vi "Wait for modem AT cmd rdy.vi"(8 "error in (no error)":errorcluster, 11 "Open serial?":bool) -> (0 "error out":errorcluster={"status"=FALSE, "code"=1073676294, "source"="VISA Read in WaitForSpecificCommResponse.vi->Wait for sierra wireless ready.vi"}, 1 "timeout?":bool, 2 "Measurement":string, 3 "Elapsed time":string)   [LabVIEW 2013]
uses:
  Test Globals/Global 1.vi
panel:
  out "Secs loop":i32
  out "Elapsed time 2":dbl=3.480198860168457
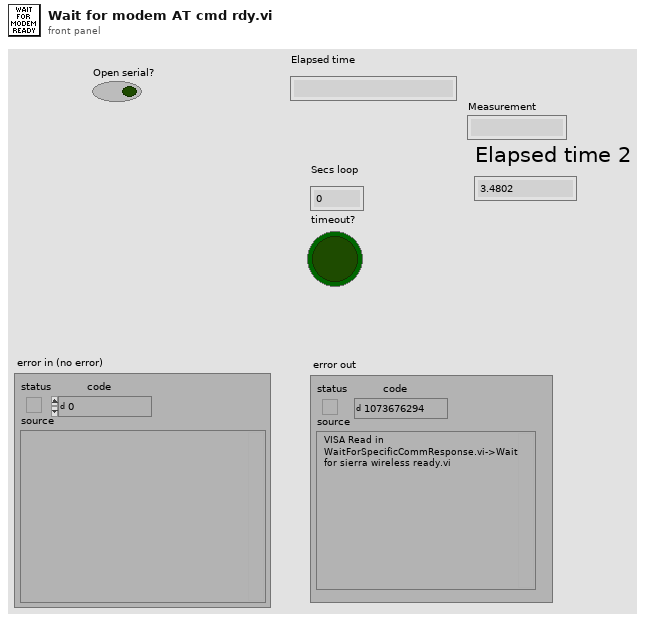
[diagram p1: front panel]
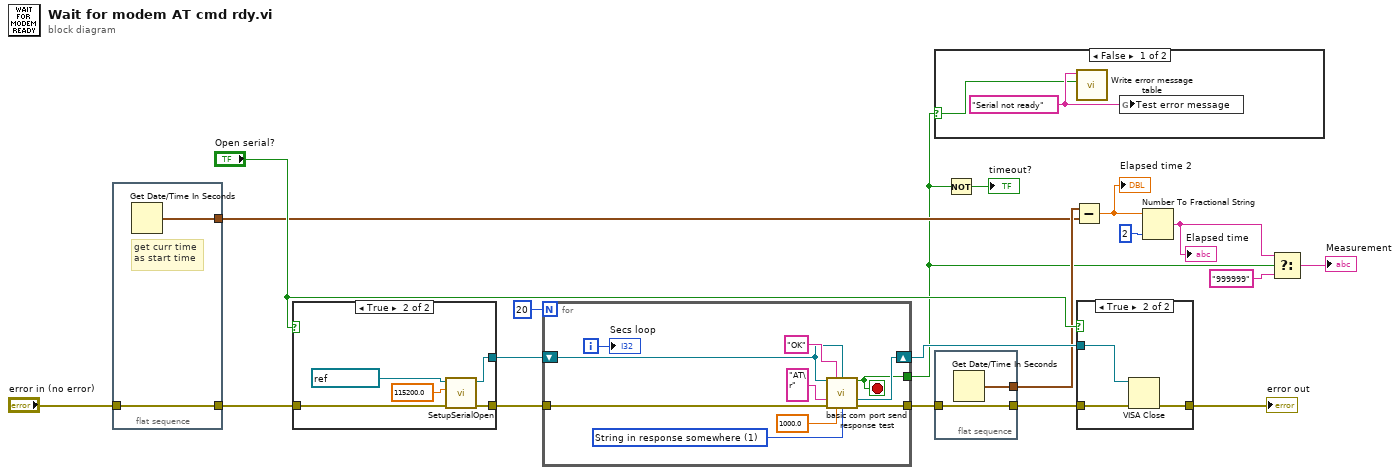
[diagram p0: block diagram]
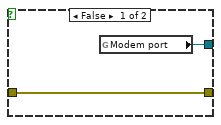
[diagram p4: hidden frame]
diagram:
  n1 = flat-sequence {
    tunnel: [w21] -> w5
    tunnel: "error in (no error)" -> [w20]
    tunnel: [w20] -> w7
    frame #0 {
      # "get curr time\nas start time"
      n2 = Get Date/Time In Seconds() -> (seconds since 1Jan1904=w21:timestamp)
    }
  }
  n3 = case shown="True" "Open serial?" {
    tunnel: w7 -> [w22 w26]
    tunnel: [w22 w25] -> w9
    tunnel: [w23 w24] -> w17
    frame False {
      n4 = global read "Global 1.vi" "Modem port"() -> (w23:refnum<visa-resource-name>)
    }
    frame True {
      n5 = call "SetupSerialOpen.vi"("error in (no error)"=w26, "Baud"=115200.0, "VISA Refnum in"=refnum<visa-resource-name> "COM30") -> ("error out"=w25:errorcluster, "VISA session"=w24:refnum<visa-resource-name>)  [unwired: 7 in]
    }
  }
  n6 = for {
    N: 20 -> [_]
    tunnel: w9 -> [w38]
    tunnel: [w33] -> w11
    tunnel: [w30] -> w2
    shift-right: [w31] -> w14
    shift-left: w17 -> [w32]
    i -> [w29]
    stop <- w30 stop-if-true
    w34 = u16 1 items=["String is exactly response", "String in response somewhere", "String not in response"] ("Comparison type")
    n7 = call "basic com port send response test.vi"("VISA Send port"=w32, "Expected response"="OK", "VISA Response Port"=w32, "Send text"="AT\r" ("write buffer"), "error in (no error)"=w38, "Wait for response msecs"=1000.0, "Comparison type"=w34) -> ("Response valid?"=w30:bool, "VISA Response Port out"=w31:refnum<visa-resource-name>, "error out"=w33:errorcluster)  [unwired: 4 in, 2 out]
    "Secs loop" <- w29
  }
  n8 = case shown="False" w2 {
    selector: w2 -> [w39 _]
    frame False {
      w40 = "Serial not ready" ("Error message)")
      n9 = call "Write error message table.vi"("Step passed?"=w39, "Error message)"=w40) -> ()  [unwired: 9 in, 1 out]
      n10 = global write "Global 1.vi" "Test error message"(w40) -> ()
    }
    frame True {
    }
  }
  n11 = flat-sequence {
    tunnel: w11 -> [w42]
    tunnel: [w42] -> w10
    tunnel: [w41] -> w6
    frame #0 {
      n12 = Get Date/Time In Seconds() -> (seconds since 1Jan1904=w41:timestamp)
    }
  }
  n13 = Not(x=w2) -> (.not. x?=→"timeout?":bool)
  n14 = Subtract(x=w6, y=w5) -> (x-y=w13:dbl)
  "Elapsed time 2" <- w13
  n15 = case shown="True" "Open serial?" {
    tunnel: [w43 w46] -> w16
    tunnel: w14 -> [_ w45]
    tunnel: w10 -> [w43 w44]
    frame False {
    }
    frame True {
      n16 = VISA Close(VISA resource name=w45, error in (no error)=w44) -> (error out=w46:errorcluster)
    }
  }
  "error out" <- w16
  n17 = Number To Fractional String(number=w13, precision (6)=i16 2) -> (F-format string=w4:string)  [unwired: 2 in]
  "Elapsed time" <- w4
  n18 = Select(t=w4, s=w2, f="999999") -> (s? t:f=→"Measurement":string)
